vi "GetSuccessors.vi"(8 "error in (no error)":errorcluster, 10 "AbstractMapNode Ref":refnum<data-value>, 11 "WorldMap in":refnum<class "NI_Robotics_DirectedGraphWorldMap.lvclass">) -> (0 "error out":errorcluster, 1 "EdgeCost":dbl[](array[numeric]), 2 "Successors":refnum<data-value>[](array[refnum]), 3 "WorldMap out":refnum<class "NI_Robotics_DirectedGraphWorldMap.lvclass">)   [LabVIEW 2017, in "NI_Robotics_DirectedGraphWorldMap.lvclass"]
uses:
  <vilib>/robotics/Navigation/shared/WorldMap/DirectedGraphWorldMap/NI_Robotics_DirectedGraphWorldMap.lvclass
  <vilib>/robotics/Navigation/shared/MapNode/AbstractMapNode/NI_Robotics_AbstractMapNode.lvclass
  <vilib>/robotics/Navigation/shared/MapNode/DirectedGraphMapNode/NI_Robotics_DirectedGraphMapNode.lvclass
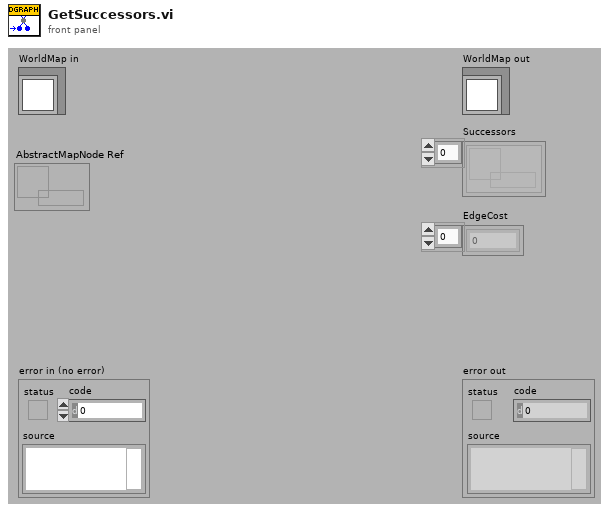
[diagram p1: front panel]
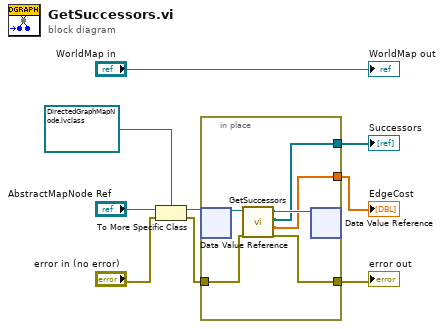
[diagram p0: block diagram]
diagram:
  n1 = To More Specific Class(target class=refnum<data-value> refnum ("data value reference"), reference="AbstractMapNode Ref", error in="error in (no error)") -> (specific class reference=w5:refnum<data-value>, error out=w2:errorcluster)
  n2 = in-place {
    in-place-border: w2 -> [w14]
    in-place-border: [w10] -> w9
    in-place-border: [w11] -> w7
    in-place-border: [w12] -> w6
    n3 = in-place-dvr #1(w5) -> (w15:refnum<class "NI_Robotics_DirectedGraphMapNode.lvclass">)  [unwired: 1 out]
    n4 = call-dynamic "GetSuccessors.vi"("error in (no error)"=w14, "DirectedGraphMapNode in"=w15) -> ("error out"=w10:errorcluster, "Successor Costs"=w12:dbl[], "Successors"=w11:refnum<data-value>[], "DirectedGraphMapNode out"=w13:refnum<class "NI_Robotics_DirectedGraphMapNode.lvclass">)  [unwired: 6 in]
    n5 = in-place-dvr #1(w13) -> ()  [unwired: 2 out]
  }
  "error out" <- w9
  "Successors" <- w7
  "EdgeCost" <- w6
  "WorldMap out" <- "WorldMap in"
